vi "Const_loop.vi"   [LabVIEW 2016]
uses:
  Instrument_Setup.vi
  Global/Global Variables/Data_Display_global.vi
  Global/Global Variables/global.vi
types:
  T1 = typedef "PSIO.ctl" = cluster{"Address":T2, "Version":enum16{"PS", "IPS"}}
  T2 = typedef "OxfordAddress.ctl" = cluster{"Com Port":i32, "ISOBUS Address":i32, "GPIB Address":i16, "Communication":enum16{"RS232", "ISOBUS", "GPIB", "Gateway"}}
  T3 = cluster{"Version\n":string, "Max Sweep(4.2K)":dbl[unit], "Max Sweep(2.2K)":dbl[unit], "Switch htr dly":dbl[unit], "Max Field(4.2K)":dbl[unit], "Max Field(2.2K)":dbl[unit], "Max lead res":dbl[unit], "IO Info":T1}
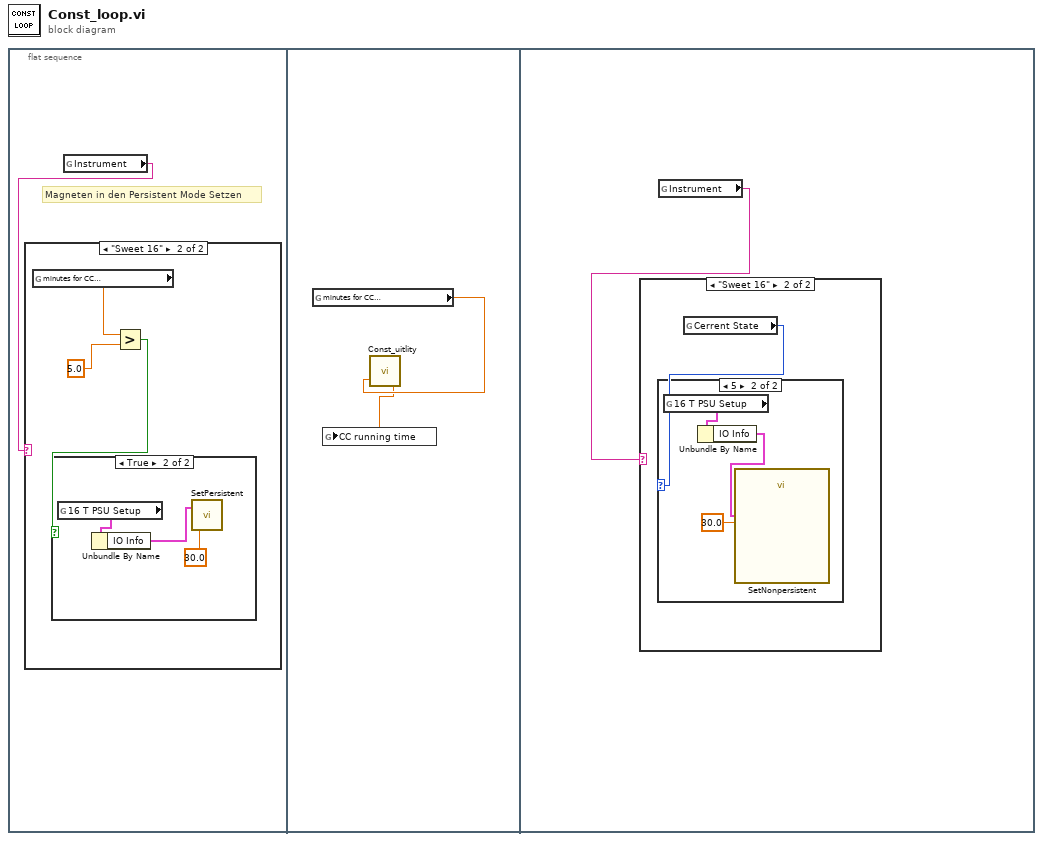
[diagram p0: block diagram]
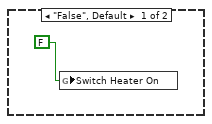
[diagram p2: hidden frame]
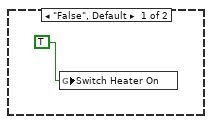
[diagram p4: hidden frame]
diagram:
  n1 = flat-sequence {
    frame #0 {
      # "Magneten in den Persistent Mode Setzen"
      n2 = global read "Instrument_Setup.vi" "Instrument"() -> (w1:string)
      n3 = case shown="\"Sweet 16\"" w1 {
        frame "False", Default {
          n4 = global write "Data_Display_global.vi" "Switch Heater On"(FALSE) -> ()
        }
        frame "Sweet 16" {
          n5 = global read "Instrument_Setup.vi" "minutes for CC\nto run"() -> (w5:dbl)
          n6 = Greater?(x=w5, y=5.0) -> (0:w3:bool)
          n7 = case shown="True" w3 {
            frame False {
            }
            frame True {
              n8 = global read "Instrument_Setup.vi" "16 T PSU Setup"() -> (w7:T3)
              n9 = Unbundle By Name(w7) -> ("IO Info"=w6:T1)
              n10 = call "SetPersistent.vi"("Switch Heater Dwell Time"=dbl[unit] 30.0, "IO Info"=w6) -> ()  [unwired: 1 in, 1 out]
            }
          }
        }
      }
    }
    frame #1 {
      n11 = global read "Instrument_Setup.vi" "minutes for CC\nto run"() -> (w10:dbl)
      n12 = call "Const_uitlity.vi"("Duration"=w10) -> ("Minutes passed"=w9:dbl)  [unwired: 1 in]
      n13 = global write "Data_Display_global.vi" "CC running time"(w9) -> ()
    }
    frame #2 {
      n14 = global read "Instrument_Setup.vi" "Instrument"() -> (w11:string)
      n15 = case shown="\"Sweet 16\"" w11 {
        frame "False", Default {
          n16 = global write "Data_Display_global.vi" "Switch Heater On"(TRUE) -> ()
        }
        frame "Sweet 16" {
          n17 = global read "global.vi" "Cerrent State"() -> (w13:i32)
          n18 = case shown="5" w13 {
            frame 0, Default {
            }
            frame 5 {
              n19 = global read "Instrument_Setup.vi" "16 T PSU Setup"() -> (w15:T3)
              n20 = Unbundle By Name(w15) -> ("IO Info"=w14:T1)
              n21 = call "SetNonpersistent.vi"("Switch Heater Dwell Time"=dbl[unit] 30.0, "IO Info"=w14) -> ()  [unwired: 2 out]
            }
          }
        }
      }
    }
  }
